vi "readVectorFile.vi"(11 "vectorFile":path) -> (2 "scalar":dbl[](array[numeric]), 3 "vectorInfo":T1 {"UVW-TI" format="%#_3g"; "XYZ-WD" format="%#_3g"})   [LabVIEW 2021]
uses:
  vectorDef.ctl
  <vilib>/Analysis/1siggen.llb/Ramp Pattern by Samples.vi
  <vilib>/Utility/file.llb/Read Delimited Spreadsheet (string).vi
  <vilib>/Analysis/NI_AALBase.lvlib
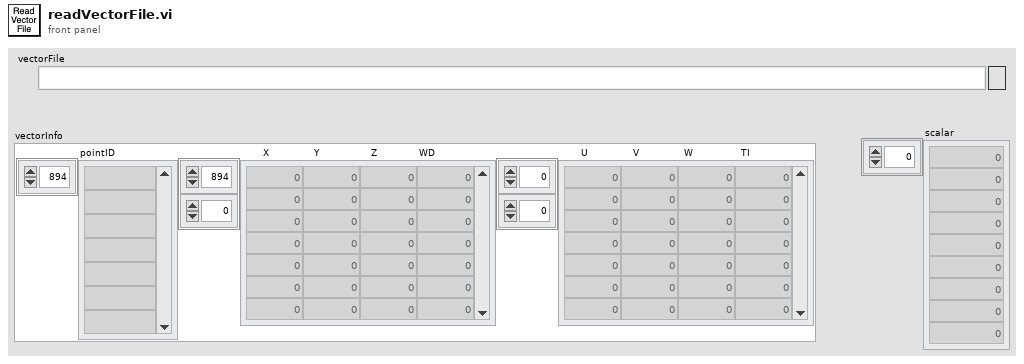
[diagram p1: front panel]
types:
  T1 = typedef "vectorDef.ctl" = cluster{"pointID":string[], "XYZ-WD":dbl[][], "UVW-TI":dbl[][]}
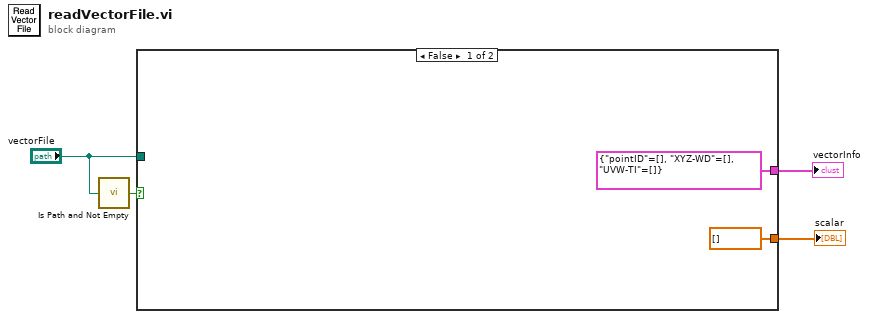
[diagram p0: block diagram]
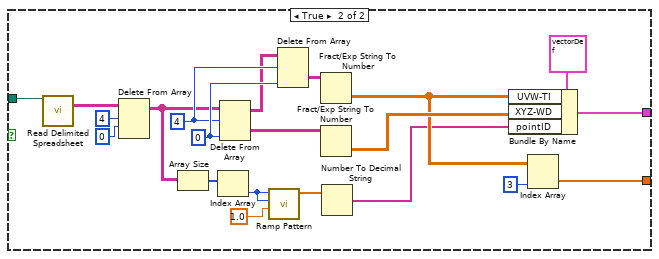
[diagram p2: hidden frame]
diagram:
  n1 = call <vilib>:"Is Path and Not Empty.vi"("path"="vectorFile") -> ("Is Path and Not Empty?"=w2:bool)  [unwired: 4 in]
  n2 = case shown="False" w2 {
    tunnel: [T1 {"pointID"=[], "XYZ-WD"=[], "UVW-TI"=[]} ("vectorInfo") w27] -> w4
    tunnel: [dbl[] [] w18] -> w3
    tunnel: "vectorFile" -> [_ w16]
    frame False {
    }
    frame True {
      w25 = 0 ("disabled index (col)")
      w20 = 4 ("length")
      n3 = call-poly <vilib>:"Read Delimited Spreadsheet.vi"("file path (dialog if empty)"=w16) -> ("all rows"=w15:string[][])  [unwired: 9 in, 5 out]
      n4 = Delete From Array(array=w15, length=4, index (row)=0) -> (array with subset deleted=w12:string[][])  [unwired: 1 in, 1 out]
      n5 = Array Size(array=w12) -> (size(s)=w11:i32[])
      n6 = Index Array(array=w11) -> (element=w7:i32)  [unwired: 1 in]
      n7 = Delete From Array(array=w12, length=w20, index (col)=w25) -> (deleted portion=w21:string[][], array with subset deleted=w19:string[][])  [unwired: 1 in]
      n8 = call-poly <vilib>:"Ramp Pattern.vi"("start"=1.0, "end"=w7, "samples"=w7) -> ("Ramp Pattern"=w9:dbl[])  [unwired: 7 in, 1 out]
      n9 = Delete From Array(array=w19, length=w20, index (col)=w25) -> (deleted portion=w22:string[][])  [unwired: 1 in, 1 out]
      n10 = Fract/Exp String To Number(string=w22) -> (number=w23:dbl[][])  [unwired: 3 in, 1 out]
      n11 = Fract/Exp String To Number(string=w21) -> (number=w24:dbl[][])  [unwired: 3 in, 1 out]
      n12 = Number To Decimal String(number=w9) -> (decimal integer string=w8:string[])  [unwired: 1 in]
      n13 = Bundle By Name(cluster=T1 {"pointID"=["1", "2", "3", "4", "5", "6", "7", "8", "9", "10", "11", "12", "13", "14", "15", "16", "17", "18", "19", "20", "21", "22", "23", "24", "25", "26", "27", "28", "29", "30", "31", "32", "33", "34", "35", "36", "37", "38", "39", "40", "41", "42", "43", "44", "45", "46", "47", "48", "49", "50", "51", "52", "53", "54", "55", "56", "57", "58", "59", "60", "61", "62", "63", "64", "65", "66", "67", "68", "69", "70", "71", "72", "73", "74", "75", "76", "77", "78", "79", "80", "81", "82", "83", "84", "85", "86", "87", "88", "89", "90", "91", "92", "93", "94", "95", "96", "97", "98", "99", "100"], "XYZ-WD"=[[-974.0, -232.0, 19.4, 0.0], [-974.0, -232.0, 29.8, 0.0], [-974.0, -232.0, 50.0, 0.0], [-974.0, -232.0, 70.2, 0.0], [-974.0, -232.0, 110.8, 0.0], [-699.0, -169.0, 110.3, 0.0], [-699.0, -169.0, 69.2, 0.0], [-699.0, -169.0, 49.1, 0.0], [-699.0, -169.0, 28.7, 0.0], [-699.0, -169.0, 18.4, 0.0], [-424.0, -105.0, 69.3, 0.0], [-424.0, -105.0, 48.5, 0.0], [-424.0, -105.0, 28.2, 0.0], [-424.0, -105.0, 18.0, 0.0], [-424.0, -105.0, 109.6, 0.0], [-450.0, 10.0, 109.9, 0.0], [-451.0, 10.0, 68.5, 0.0], [-451.0, 10.0, 48.1, 0.0], [-451.0, 10.0, 27.9, 0.0], [-451.0, 10.0, 17.6, 0.0], [-479.0, 135.0, 68.5, 0.0], [-479.0, 135.0, 47.8, 0.0], [-479.0, 135.0, 27.5, 0.0], [-479.0, 135.0, 17.3, 0.0], [-479.0, 135.0, 109.0, 0.0], [-212.0, 196.0, 109.1, 0.0], [-212.0, 196.0, 67.8, 0.0], [-212.0, 196.0, 47.3, 0.0], [-212.0, 196.0, 27.0, 0.0], [-212.0, 196.0, 16.9, 0.0], [-183.0, 72.0, 68.1, 0.0], [-184.0, 72.0, 47.3, 0.0], [-184.0, 72.0, 27.0, 0.0], [-184.0, 72.0, 16.9, 0.0], [-184.0, 72.0, 108.5, 0.0], [-157.0, -44.0, 109.5, 0.0], [-157.0, -44.0, 68.4, 0.0], [-157.0, -44.0, 48.2, 0.0], [-157.0, -44.0, 27.9, 0.0], [-157.0, -44.0, 17.7, 0.0], [111.0, 18.0, 68.4, 0.0], [110.0, 18.0, 47.8, 0.0], [110.0, 18.0, 27.4, 0.0], [110.0, 18.0, 17.2, 0.0], [110.0, 18.0, 108.9, 0.0], [84.0, 133.0, 109.2, 0.0], [84.0, 133.0, 67.7, 0.0], [84.0, 133.0, 47.3, 0.0], [84.0, 133.0, 27.1, 0.0], [84.0, 133.0, 16.9, 0.0], [55.0, 258.0, 67.6, 0.0], [55.0, 258.0, 46.9, 0.0], [55.0, 258.0, 26.7, 0.0], [55.0, 258.0, 16.4, 0.0], [55.0, 258.0, 108.2, 0.0], [274.0, 326.0, 107.9, 0.0], [274.0, 325.0, 66.9, 0.0], [274.0, 325.0, 46.5, 0.0], [274.0, 325.0, 26.1, 0.0], [274.0, 325.0, 16.0, 0.0], [309.0, 170.0, 67.7, 0.0], [309.0, 170.0, 46.8, 0.0], [309.0, 170.0, 26.6, 0.0], [309.0, 170.0, 16.4, 0.0], [309.0, 170.0, 108.1, 0.0], [333.0, 68.0, 108.3, 0.0], [333.0, 69.0, 67.3, 0.0], [333.0, 69.0, 46.9, 0.0], [333.0, 69.0, 26.8, 0.0], [333.0, 69.0, 16.4, 0.0], [560.0, 121.0, 67.3, 0.0], [560.0, 121.0, 46.6, 0.0], [560.0, 121.0, 26.1, 0.0], [560.0, 121.0, 16.1, 0.0], [560.0, 121.0, 107.7, 0.0], [537.0, 222.0, 107.9, 0.0], [537.0, 222.0, 66.8, 0.0], [537.0, 222.0, 46.7, 0.0], [537.0, 222.0, 26.1, 0.0], [537.0, 222.0, 16.1, 0.0], [502.0, 378.0, 67.3, 0.0], [501.0, 378.0, 46.5, 0.0], [501.0, 378.0, 26.3, 0.0], [501.0, 378.0, 16.0, 0.0], [501.0, 378.0, 107.6, 0.0], [729.0, 430.0, 107.8, 0.0], [729.0, 430.0, 66.9, 0.0], [729.0, 430.0, 46.5, 0.0], [729.0, 430.0, 26.2, 0.0], [729.0, 430.0, 16.0, 0.0], [765.0, 275.0, 67.3, 0.0], [765.0, 275.0, 46.5, 0.0], [765.0, 275.0, 26.1, 0.0], [765.0, 275.0, 16.1, 0.0], [765.0, 275.0, 107.6, 0.0], [788.0, 173.0, 107.8, 0.0], [788.0, 173.0, 67.3, 0.0], [788.0, 173.0, 46.9, 0.0], [788.0, 173.0, 26.7, 0.0], [788.0, 173.0, 16.3, 0.0]], "UVW-TI"=[[0.507, -0.018, -0.012, 19.0], [0.588, -0.005, 0.006, 18.0], [0.64, -0.014, 0.003, 18.0], [0.699, -0.006, 0.002, 16.0], [0.749, -0.015, 0.003, 14.0], [0.722, -0.003, 0.0, 16.0], [0.672, -0.011, 0.006, 16.0], [0.626, -0.012, 0.01, 17.0], [0.579, -0.012, 0.004, 17.0], [0.483, -0.013, 0.0, 19.0], [0.657, -0.017, 0.001, 17.0], [0.608, -0.015, 0.0, 19.0], [0.535, -0.01, 0.0, 18.0], [0.474, -0.002, -0.007, 20.0], [0.707, -0.011, 0.001, 15.0], [0.719, -0.007, -0.001, 15.0], [0.671, -0.023, -0.006, 16.0], [0.609, -0.027, -0.003, 18.0], [0.528, -0.025, -0.009, 19.0], [0.441, -0.011, -0.001, 21.0], [0.688, -0.02, -0.006, 16.0], [0.641, -0.03, -0.006, 17.0], [0.531, -0.026, -0.016, 19.0], [0.402, -0.007, -0.008, 22.0], [0.726, -0.011, -0.007, 14.0], [0.735, -0.009, -0.004, 13.0], [0.687, -0.009, -0.005, 15.0], [0.654, -0.004, -0.002, 16.0], [0.609, -0.01, 0.002, 16.0], [0.553, -0.013, 0.009, 17.0], [0.704, -0.015, -0.001, 15.0], [0.648, -0.017, 0.0, 17.0], [0.582, -0.026, 0.007, 17.0], [0.533, -0.026, 0.013, 19.0], [0.736, -0.01, 0.001, 13.0], [0.738, -0.013, 0.0, 14.0], [0.685, -0.015, 0.001, 15.0], [0.645, -0.016, 0.001, 17.0], [0.579, -0.019, -0.001, 18.0], [0.511, -0.011, -0.006, 18.0], [0.707, -0.002, -0.003, 15.0], [0.649, -0.012, 0.0, 17.0], [0.61, -0.013, -0.003, 17.0], [0.565, -0.009, -0.008, 17.0], [0.735, -0.011, -0.001, 15.0], [0.727, -0.007, 0.006, 16.0], [0.663, -0.011, 0.01, 17.0], [0.643, -0.015, 0.015, 17.0], [0.588, -0.027, 0.012, 18.0], [0.532, -0.027, 0.006, 18.0], [0.668, -0.01, 0.004, 18.0], [0.625, -0.014, 0.007, 19.0], [0.6, -0.031, 0.008, 19.0], [0.535, -0.019, -0.001, 20.0], [0.731, -0.01, 0.002, 16.0], [0.759, -0.009, -0.005, 13.0], [0.723, -0.008, -0.002, 14.0], [0.703, -0.014, -0.002, 14.0], [0.67, -0.007, 0.0, 14.0], [0.627, -0.007, -0.008, 16.0], [0.702, -0.018, -0.003, 14.0], [0.671, -0.022, -0.003, 17.0], [0.638, -0.035, -0.005, 17.0], [0.554, -0.031, -0.018, 18.0], [0.753, -0.008, -0.004, 15.0], [0.725, -0.007, 0.004, 15.0], [0.675, -0.013, 0.003, 16.0], [0.648, -0.015, -0.003, 17.0], [0.533, -0.004, -0.013, 20.0], [0.471, 0.003, -0.002, 22.0], [0.722, -0.002, 0.007, 13.0], [0.695, 0.0, 0.008, 14.0], [0.648, 0.002, 0.003, 15.0], [0.611, 0.005, -0.006, 16.0], [0.761, -0.007, 0.003, 13.0], [0.758, -0.009, -0.001, 13.0], [0.741, -0.009, -0.001, 13.0], [0.711, -0.005, 0.002, 14.0], [0.679, -0.003, -0.002, 15.0], [0.629, -0.003, -0.007, 15.0], [0.738, -0.01, -0.001, 13.0], [0.716, -0.003, -0.001, 14.0], [0.68, -0.001, -0.001, 14.0], [0.627, -0.003, -0.003, 15.0], [0.764, -0.003, -0.004, 13.0], [0.777, -0.008, -0.002, 12.0], [0.747, -0.008, 0.003, 13.0], [0.723, -0.01, 0.002, 13.0], [0.688, -0.009, -0.001, 14.0], [0.649, -0.012, -0.004, 16.0], [0.763, 0.0, 0.001, 13.0], [0.722, -0.004, 0.005, 13.0], [0.679, -0.004, 0.001, 15.0], [0.643, 0.001, 0.0, 16.0], [0.782, -0.003, 0.0, 12.0], [0.788, -0.009, 0.002, 11.0], [0.741, -0.001, 0.0, 13.0], [0.721, -0.003, 0.004, 13.0], [0.69, 0.004, 0.001, 14.0], [0.641, 0.001, -0.004, 15.0]]} ("vectorInfo"), "UVW-TI"=w23, "XYZ-WD"=w24, "pointID"=w8) -> (w27:T1)
      n14 = Index Array(array=w23, index (col)=3 ("disabled index (col)")) -> (element=w18:dbl[])  [unwired: 1 in]
    }
  }
  "vectorInfo" <- w4
  "scalar" <- w3
